vi "Get Last Time.vi"(8 "error in (no error)":errorcluster, 11 "[MV] Key Certify in":refnum<class "[MV] Key Certify.lvclass">) -> (0 "error out":errorcluster, 3 "[MV] Key Certify out":refnum<class "[MV] Key Certify.lvclass">)   [LabVIEW 2020, in "[MV] Key Certify.lvlib" / "[MV] Key Certify.lvclass"]
uses:
  [MV] Key Certify.lvclass
  <vilib>/registry/registry.llb/Registry RtKey.ctl
  <vilib>/registry/registry.llb/Read Registry Value Simple STR.vi
  <vilib>/YU/YU-Template/Time/SubVI/Single String(s) to Stamp.vi
  <vilib>/registry/registry.llb/Write Registry Value Simple STR.vi
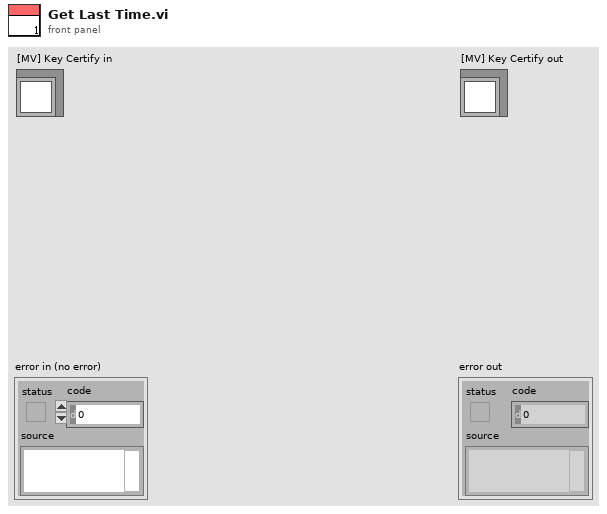
[diagram p1: front panel]
types:
  T1 = typedef "Registry RtKey.ctl" = enum32{"HKEY_CLASSES_ROOT", "HKEY_CURRENT_USER", "HKEY_LOCAL_MACHINE", "HKEY_USERS", "HKEY_PERFORMANCE_DATA", "HKEY_CURRENT_CONFIG", "HKEY_DYN_DATA"}
  T2 = typedef "Registry refnum.ctl" = refnum<k1>
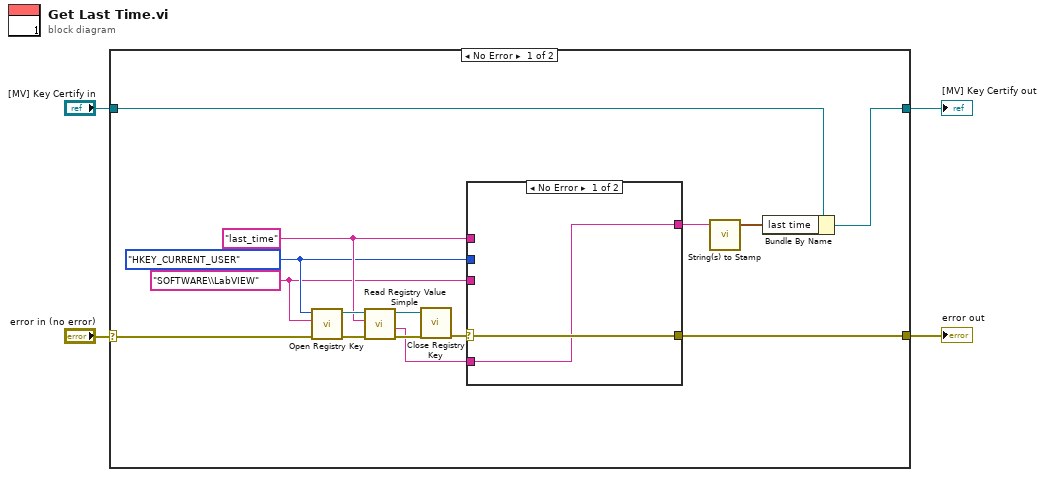
[diagram p0: block diagram]
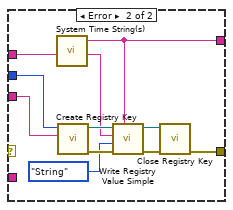
[diagram p2: hidden frame]
diagram:
  n1 = case shown="No Error" "error in (no error)" {
    selector: "error in (no error)" -> [w19 w33]
    tunnel: [w9 w33] -> w3
    tunnel: [w5 w32] -> w1
    tunnel: "[MV] Key Certify in" -> [w7 w32]
    frame No Error {
      w13 = "last_time" ("String/Binary data")
      w12 = Registry_RtKey."HKEY_CURRENT_USER" ("root key (HKEY_LOCAL_MACHINE)")
      w11 = "SOFTWARE\\LabVIEW" ("subkey")
      n2 = call <vilib>:"Open Registry Key.vi"("error in (no error)"=w19, "subkey"=w11, "root key (HKEY_LOCAL_MACHINE)"=w12) -> ("error out"=w18:errorcluster, "refnum out"=w17:T2)  [unwired: 7 in]
      n3 = call-poly <vilib>:"Read Registry Value Simple.vi"("error in (no error)"=w18, "value"=w13, "refnum"=w17) -> ("error out"=w15:errorcluster, "String/Binary data"=w10:string, "refnum out"=w16:T2)  [unwired: 3 in, 1 out]
      n4 = call <vilib>:"Close Registry Key.vi"("error in (no error)"=w15, "refnum"=w16) -> ("error out"=w14:errorcluster)  [unwired: 5 in]
      n5 = case shown="No Error" w14 {
        selector: w14 -> [w21 _]
        tunnel: w13 -> [_ w27]
        tunnel: w12 -> [_ w26]
        tunnel: w11 -> [_ w25]
        tunnel: [w20 w24] -> w8
        tunnel: w10 -> [w20 _]
        tunnel: [w21 w23] -> w9
        frame No Error {
        }
        frame Error {
          n6 = call <vilib>:"System Time String(s).vi"() -> ("system time string(s)"=w24:string)  [unwired: 5 in]
          n7 = call <vilib>:"Create Registry Key.vi"("subkey"=w25, "root key (HKEY_LOCAL_MACHINE)"=w26) -> ("error out"=w31:errorcluster, "refnum out"=w30:T2)  [unwired: 7 in, 1 out]
          n8 = call-poly <vilib>:"Write Registry Value Simple.vi"("String/Binary data"=w24, "error in (no error)"=w31, "simple data type"=enum16{"String", "Binary", "DWORD"}."String", "value"=w27, "refnum"=w30) -> ("error out"=w29:errorcluster, "refnum out"=w28:T2)  [unwired: 3 in]
          n9 = call <vilib>:"Close Registry Key.vi"("error in (no error)"=w29, "refnum"=w28) -> ("error out"=w23:errorcluster)  [unwired: 5 in]
        }
      }
      n10 = call-poly <vilib>:"String(s) to Stamp.vi"("time string(ms)"=w8) -> ("time stamp(ms)"=w6:timestamp)  [unwired: 4 in]
      n11 = Bundle By Name(cluster=w7, "last time"=w6) -> (w5:refnum<class "[MV] Key Certify.lvclass">)
    }
    frame Error {
    }
  }
  "error out" <- w3
  "[MV] Key Certify out" <- w1
